vi "RelativeHumidity.vi"(0 "DewPoint_T In":sgl, 1 "StackIn_T In":sgl, 2 "RH(%) In":sgl, 3 "OptionList":enum16{"DewPoint_T(℃)", "StackIn_T(℃)", "RH(%)"}(ring)) -> (7 "DewPoint_T Out":sgl, 8 "StackIn_T Out":sgl, 9 "RH(%) Out":sgl)   [LabVIEW 2020]
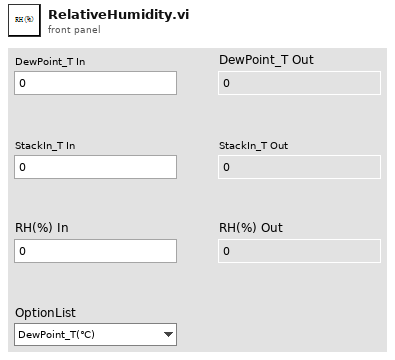
[diagram p1: front panel]
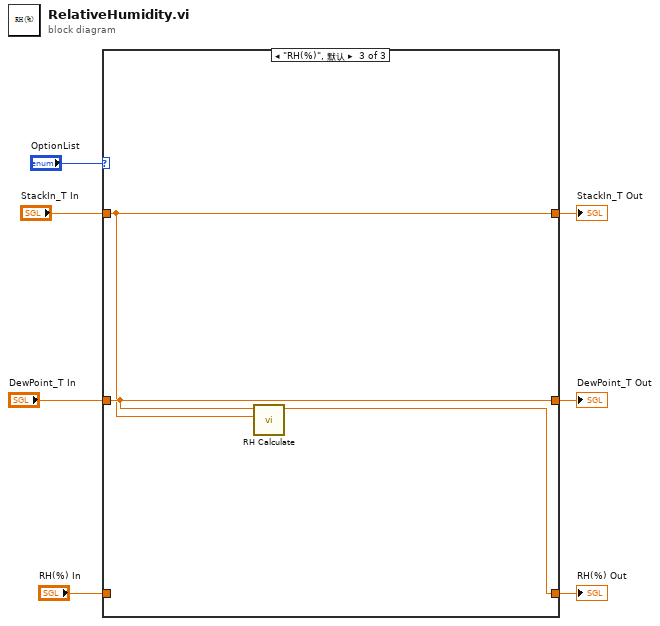
[diagram p0: block diagram]
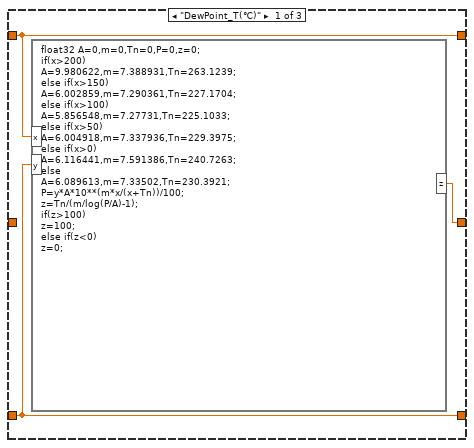
[diagram p2: hidden frame]
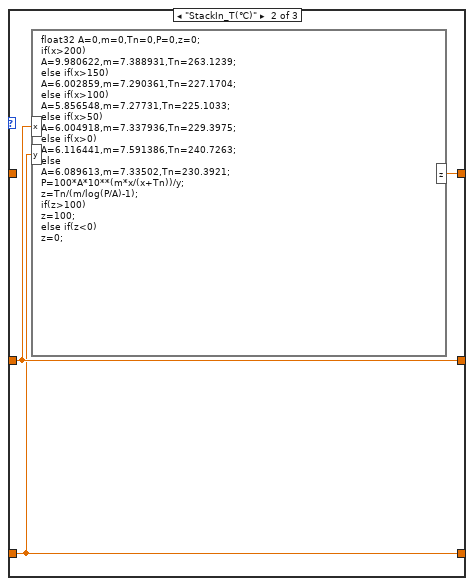
[diagram p3: hidden frame]
diagram:
  n1 = case shown="\"RH(%)\", 默认" "OptionList" {
    tunnel: "RH(%) In" -> [w8 w11 _]
    tunnel: "StackIn_T In" -> [w9 _ w15]
    tunnel: "DewPoint_T In" -> [_ w12 w16]
    tunnel: [w10 w12 w16] -> w6
    tunnel: [w9 w13 w15] -> w2
    tunnel: [w8 w11 w14] -> w1
    frame "DewPoint_T(℃)" {
      n2 = formula code="float32 A=0,m=0,Tn=0,P=0,z=0;\nif(x>200)\nA=9.980622,m=7.388931,Tn=263.1239;\nelse if(x>150)\nA=6.002859,m=7.290361,Tn=227.1704;\nelse if(x>100)\nA=5.856548,m=7.27731,Tn=225.1033;\nelse if(x>50)\nA=6.004918,m=7.337936,Tn=229.3975;\nelse if(x>0)\nA=6.116441,m=7.591386,Tn=240.7263;\nelse\nA=6.089613,m=7.33502,Tn=230.3921;\nP=y*A*10**(m*x/(x+Tn))/100;\nz=Tn/(m/log(P/A)-1);\nif(z>100)\nz=100;\nelse if(z<0)\nz=0;"("x"=w9, "y"=w8) -> ("z"=w10:sgl)
    }
    frame "StackIn_T(℃)" {
      n3 = formula code="float32 A=0,m=0,Tn=0,P=0,z=0;\nif(x>200)\nA=9.980622,m=7.388931,Tn=263.1239;\nelse if(x>150)\nA=6.002859,m=7.290361,Tn=227.1704;\nelse if(x>100)\nA=5.856548,m=7.27731,Tn=225.1033;\nelse if(x>50)\nA=6.004918,m=7.337936,Tn=229.3975;\nelse if(x>0)\nA=6.116441,m=7.591386,Tn=240.7263;\nelse\nA=6.089613,m=7.33502,Tn=230.3921;\nP=100*A*10**(m*x/(x+Tn))/y;\nz=Tn/(m/log(P/A)-1);\nif(z>100)\nz=100;\nelse if(z<0)\nz=0;"("x"=w12, "y"=w11) -> ("z"=w13:sgl)
    }
    frame "RH(%)", Default {
      n4 = call "RH Calculate.vi"("T_饱和"=w15, "T_露点"=w16) -> ("RH(%)"=w14:sgl)  [unwired: 7 in, 2 out]
    }
  }
  "DewPoint_T Out" <- w6
  "StackIn_T Out" <- w2
  "RH(%) Out" <- w1
